vi "setUp.vi"(8 "error in (no error)":errorcluster, 11 "reference in":refnum<class "TestCSMSuite.lvclass">) -> (0 "error out":errorcluster, 3 "reference out":refnum<class "TestCSMSuite.lvclass">)   [LabVIEW 2017, in "TestCSMSuite.lvclass"]
doc: "setUp runs prior to the test method during test execution. Use this method to initialize any object data required by your tests."
uses:
  TestCSMSuite.lvclass
  C:/Program Files (x86)/National Instruments/LabVIEW 2017/vi.lib/addons/_JKI Toolkits/VI Tester/TestSuite.llb/TestSuite.lvclass
  <vilib>/addons/_JKI Toolkits/VI Tester/TestSuite.llb/TestSuite.lvclass
  src/user.lib/_NEVSTOP/Communicable State Machine(CSM)/addons/Logger/CSM File Logger.lvlib
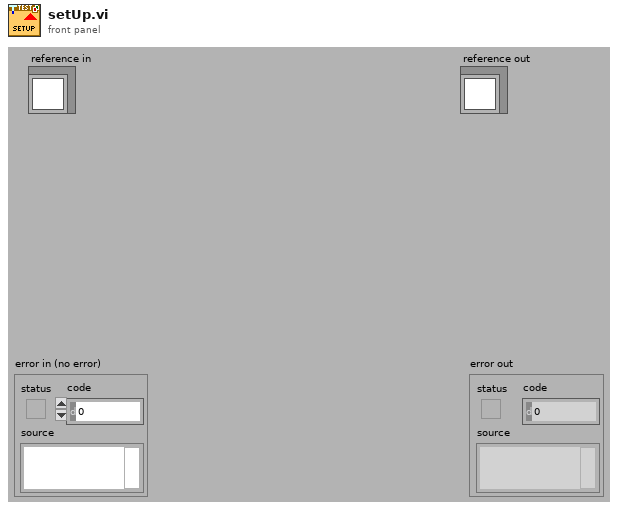
[diagram p1: front panel]
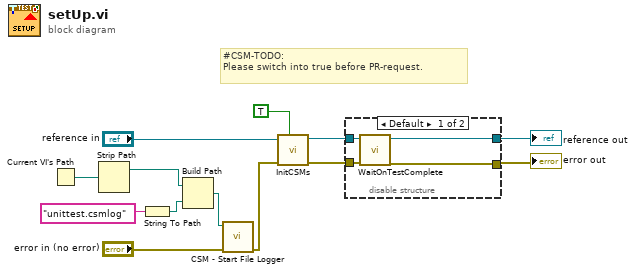
[diagram p0: block diagram]
diagram:
  # "#CSM-TODO:\nPlease switch into true before PR-request."
  n1 = Current VI's Path() -> (path=w5:path)
  n2 = Strip Path(path=w5) -> (stripped path=w2:path)  [unwired: 1 out]
  n3 = String To Path(string="unittest.csmlog") -> (path=w3:path)
  n4 = Build Path(base path=w2, name or relative path=w3) -> (appended path=w1:path)
  n5 = call "CSM - Start File Logger.vi"("Error In"="error in (no error)", "Log File Path"=w1) -> ("error out"=w6:errorcluster)  [unwired: 7 in, 2 out]
  n6 = call "InitCSMs.vi"("Enable Conditional Building lvlibp?"=TRUE, "error in"=w6, "TestCSMSuite in"="reference in") -> ("error out"=w9:errorcluster, "TestCSMSuite out"=w10:refnum<class "TestCSMSuite.lvclass">)  [unwired: 7 in]
  n7 = disable-structure shown="Default" {
    disable-tunnel: w10 -> [w17 w18]
    disable-tunnel: [w16 w18] -> w13
    disable-tunnel: w9 -> [w15 w19]
    disable-tunnel: [w14 w19] -> w12
    frame condition #0 (active) {
      n8 = call <vilib>:"WaitOnTestComplete.vi"("error in (no error)"=w15, "TestSuite in"=w17) -> ("error out"=w14:errorcluster, "TestSuite out"=w16:refnum<class "TestCSMSuite.lvclass">)  [unwired: 8 in]
    }
    frame condition #1 {
    }
  }
  "error out" <- w12
  "reference out" <- w13
